vi "3.vi"() -> ()   [LabVIEW 2017]
panel:
  out "数组":dbl[][](array[numeric])
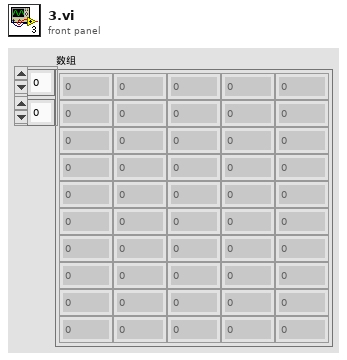
[diagram p1: front panel]
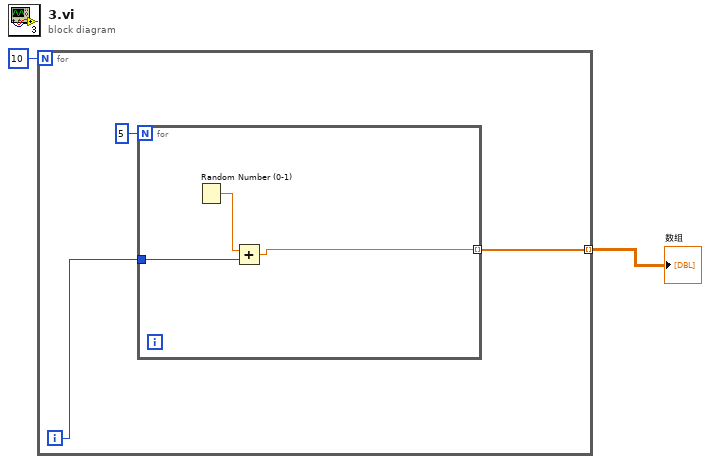
[diagram p0: block diagram]
diagram:
  n1 = for {
    N: 10 -> [_]
    tunnel: [w3] -> w1 mode=indexing
    i -> [w4]
    n2 = for {
      N: 5 -> [_]
      tunnel: w4 -> [w7]
      tunnel: [w6] -> w3 mode=indexing
      n3 = Random Number (0-1)() -> (number: 0 to 1=w8:dbl)
      n4 = Add(x=w8, y=w7) -> (x+y=w6:dbl)
    }
  }
  "数组" <- w1
